vi "RUS Sweep -- build content of txt file.vi"(7 "temperature boxes":T1={"LTC21 Address"="GPIB0::15::INSTR", "ITC503 Address"="GPIB0::24::INSTR", "ITC temperature"=299.2, "ITC set temperature"=295.0, "LTC temperature"=0.0, "heater"=0.0, "gas flow"=90.0, "P"=10.0, "D"=1.0, "I"=3.0, "ITC state"="X0A1C2S00H1L0\r", "nonzero temperature"=0.0, "Magn Field (T)"=0.0, "LakeShore340"="", "LS340 Adress"=0, "Sample Temperature Source"=enum."read T <- LakeShore 340", "Neocera sensor"=1}, 8 "error in":errorcluster, 9 "Column Names (\\t for TAB)":string="Frequency\\tX\\tY", 10 "thermometer snapshot":T5={"ITC Temperature"=0.0, "ITC Set Temperature"=0.0, "LTC Temperature"=0.0, "LTC21 Address"="GPIB0::15::INSTR", "ITC503 Address"="GPIB0::24::INSTR"}, 11 "Save data settings":T3={"Save data"=TRUE, "Data Root Path"=path "", "File Prefix"="", "File Format"=enum."ASCII", "Save column names"=TRUE, "File Comments"="<Description of the current file>", "User/Prj"="<User Name/Project Description>"}) -> (0 "error out":errorcluster={"status"=TRUE, "code"=-200019, "source"="DAQmx Read (Analog 1D Wfm NChan NSamp).vi:1<append>\n<B>Task Name: </B>_unnamedTask<2C36>"}, 3 "Save data settings out":T3={"Save data"=TRUE, "Data Root Path"=path "", "File Prefix"="", "File Format"=enum."ASCII", "Save column names"=TRUE, "File Comments"="<Description of the current file>", "User/Prj"="<User Name/Project Description>"})   [LabVIEW 2015]
uses:
  NHMFL_Core/Libraries/File/Controls/Save data settings.ctl
  NHMFL_Core/Libraries/File/Controls/File formats.ctl
  state.ctl
  Sample_Temperature_Source_Control.ctl
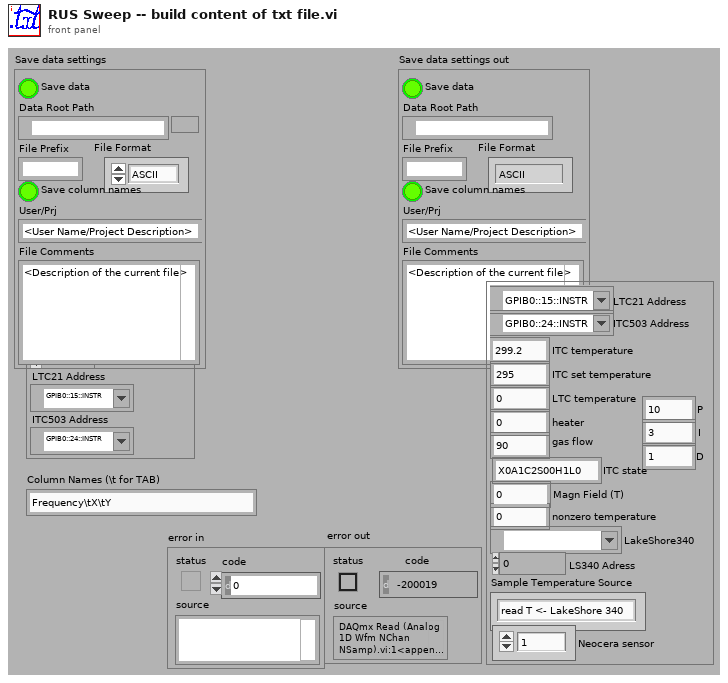
[diagram p1: front panel]
types:
  T1 = typedef "state.ctl" = cluster{"LTC21 Address":refnum<visa-resource-name>, "ITC503 Address":refnum<visa-resource-name>, "ITC temperature":dbl, "ITC set temperature":dbl, "LTC temperature":dbl, "heater":dbl, "gas flow":dbl, "P":dbl, "D":dbl, "I":dbl, "ITC state":string, "nonzero temperature":dbl, "Magn Field (T)":dbl, "LakeShore340":refnum<visa-resource-name>, "LS340 Adress":i16, "Sample Temperature Source":T2, "Neocera sensor":i32}
  T2 = typedef "Sample_Temperature_Source_Control.ctl" = enum16{"read T <- LakeShore 340", "read T <- Neocera"}
  T3 = typedef "Save data settings.ctl" = cluster{"Save data":bool, "Data Root Path":path, "File Prefix":string, "File Format":T4, "Save column names":bool, "File Comments":string, "User/Prj":string}
  T4 = typedef "File formats.ctl" = enum16{"TDMS", "ASCII", "BINARY"}
  T5 = cluster{"ITC Temperature":dbl, "ITC Set Temperature":dbl, "LTC Temperature":dbl, "LTC21 Address":refnum<visa-resource-name>, "ITC503 Address":refnum<visa-resource-name>}
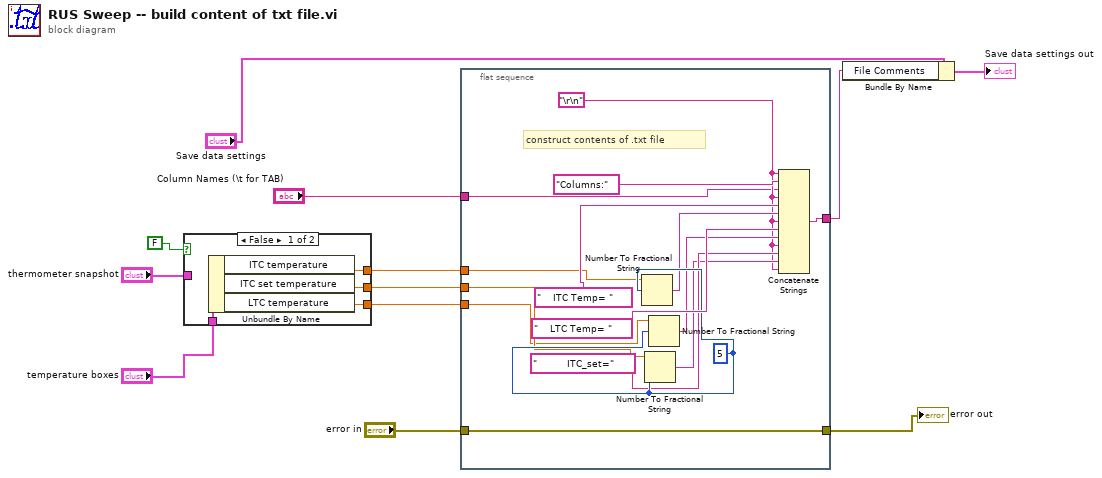
[diagram p0: block diagram]
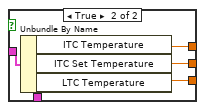
[diagram p2: hidden frame]
diagram:
  n1 = case shown="False" FALSE {
    tunnel: "thermometer snapshot" -> [_ w20]
    tunnel: [w16 w19] -> w9
    tunnel: [w15 w18] -> w8
    tunnel: [w14 w17] -> w7
    tunnel: "temperature boxes" -> [w13 _]
    frame False {
      n2 = Unbundle By Name(w13) -> ("ITC temperature"=w16:dbl, "ITC set temperature"=w15:dbl, "LTC temperature"=w14:dbl)
    }
    frame True {
      n3 = Unbundle By Name(w20) -> ("ITC Temperature"=w19:dbl, "ITC Set Temperature"=w18:dbl, "LTC Temperature"=w17:dbl)
    }
  }
  n4 = flat-sequence {
    tunnel: [w26] -> w3
    tunnel: [w25] -> w12
    tunnel: "error in" -> [w25]
    tunnel: w9 -> [w24]
    tunnel: w8 -> [w23]
    tunnel: w7 -> [w22]
    tunnel: "Column Names (\\t for TAB)" -> [w21]
    frame #0 {
      w33 = i16 5 ("width (-)")
      w27 = "\r\n"
      # "construct contents of .txt file"
      n5 = Number To Fractional String(number=w24, width (-)=w33) -> (F-format string=w31:string)  [unwired: 2 in]
      n6 = Number To Fractional String(number=w23, precision (6)=w33) -> (F-format string=w28:string)  [unwired: 2 in]
      n7 = Number To Fractional String(number=w22, width (-)=w33) -> (F-format string=w30:string)  [unwired: 2 in]
      n8 = Concatenate Strings(w27, "Columns:", w21, w27, "    ITC Temp= " ("string"), w31, w27, "    LTC Temp= " ("string"), w30, w27, "          ITC_set=" ("string"), w28, w27) -> (w26:string)
    }
  }
  n9 = Bundle By Name(cluster="Save data settings", "File Comments"=w3) -> (→"Save data settings out":T3)
  "error out" <- w12
